vi "load_cells.vi"() -> ()   [LabVIEW 2020]
uses:
  <vilib>/ULx/Create Channel.llb/ULx Create Channel (AI-Voltage-Basic).vi
  <vilib>/ULx/Timing.llb/ULx Timing (Sample Clock).vi
  <vilib>/ULx/Read.llb/ULx Read (Analog 1D Wfm NChan NSamp).vi
panel:
  out "Waveform Graph":waveform(dbl)[](graph)
  in  "rate":dbl=1000.0
  in  "samples per channel":i32=1000
  in  "sample mode":i32(ring) items=["FiniteSamples", "ContinuousSamples"]
  in  "minimum value":dbl=-5.0
  in  "maximum value":dbl=5.0
  in  "physical channels":refnum<k21>
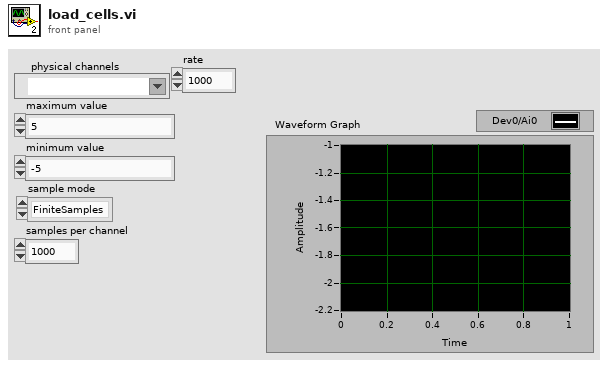
[diagram p1: front panel]
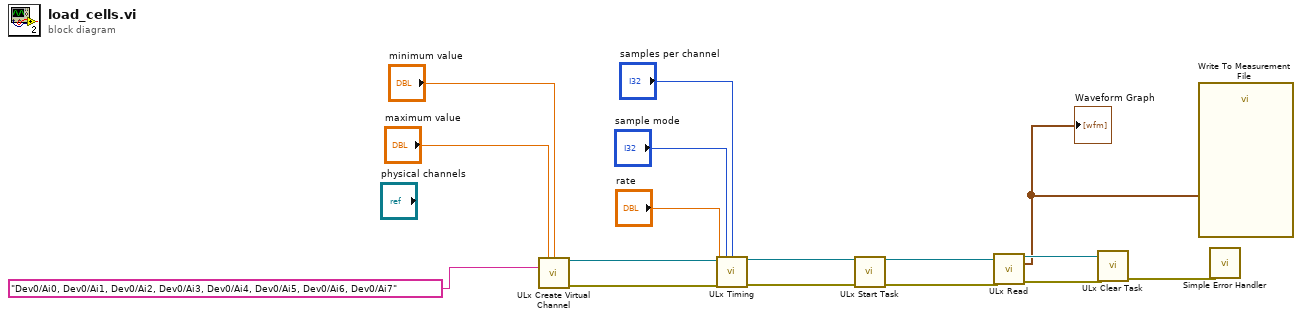
[diagram p0: block diagram]
diagram:
  n1 = call-poly <vilib>:"ULx Create Virtual Channel.vi"("maximum value"="maximum value", "minimum value"="minimum value", "physical channels"="Dev0/Ai0, Dev0/Ai1, Dev0/Ai2, Dev0/Ai3, Dev0/Ai4, Dev0/Ai5, Dev0/Ai6, Dev0/Ai7") -> ("task out"=w11:refnum<k24>, "error out"=w10:errorcluster)  [unwired: 11 in]
  n2 = call-poly <vilib>:"ULx Timing.vi"("task in"=w11, "sample mode"="sample mode", "samples per channel"="samples per channel", "rate"="rate", "error in"=w10) -> ("task out"=w9:refnum<k24>, "error out"=w8:errorcluster)  [unwired: 9 in]
  n3 = call <vilib>:"ULx Start Task.vi"("task in"=w9, "error in"=w8) -> ("task out"=w6:refnum<k24>, "error out"=w7:errorcluster)  [unwired: 12 in]
  n4 = call-poly <vilib>:"ULx Read.vi"("task in"=w6, "error in"=w7) -> ("task out"=w4:refnum<k24>, "data"=w2:waveform(dbl)[], "error out"=w5:errorcluster)  [unwired: 11 in]
  "Waveform Graph" <- w2
  n5 = call <vilib>:"ULx Clear Task.vi"("task in"=w4, "error in"=w5) -> ("error out"=w3:errorcluster)  [unwired: 13 in]
  n6 = call "Write To Measurement File"("Signals"=w2) -> ()  [unwired: 16 in, 3 out]
  n7 = call <vilib>:"Simple Error Handler.vi"("error in (no error)"=w3) -> ()  [unwired: 4 in, 5 out]
